vi "GlobalValues.vi"() -> ()   [LabVIEW 2023]
panel:
  in  "secondHour":dbl=10.2
  in  "firstHour":dbl=12.5
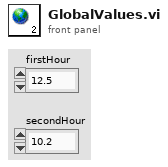
[diagram p1: front panel]
diagram:
